vi "Initialize With Options.vi"(7 "option string":string, 8 "error in (no error)":errorcluster {"code" format="%.0x"}, 9 "reset device (Off)":bool, 10 "id query (Off)":bool, 11 "resource string":string caption="resource name") -> (0 "error out":errorcluster {"code" format="%.0x"}, 3 "instrument handle out":refnum<k15>)   [LabVIEW 2014, in "Agilent NA.lvlib"]
doc: "Opens the I/O session to the instrument. Driver methods and properties that access the instrument are only accessible after Initialize is called. Initialize optionally performs a Reset and queries the instrument to validate the instrument model."
uses:
  Agilent NA.lvlib
  AgNA.dll
panel:
  # "© 2014 Agilent Technologies, Inc."
  # "© 2000-2008 National Instruments.  All Rights Reserved."
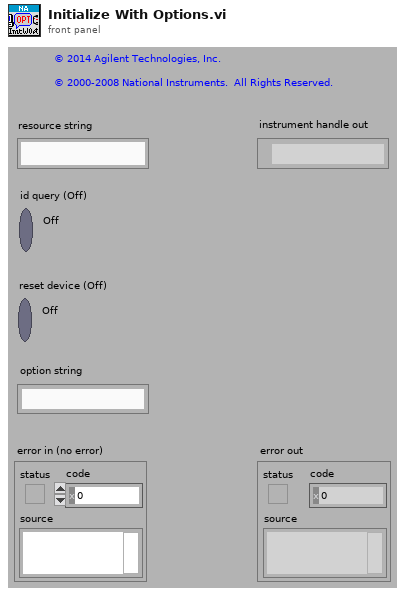
[diagram p1: front panel]
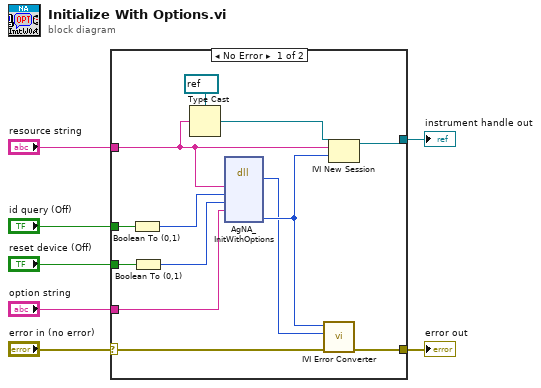
[diagram p0: block diagram]
diagram:
  n1 = case shown="No Error" "error in (no error)" {
    selector: "error in (no error)" -> [w12 w22]
    tunnel: [w11 w22] -> w6
    tunnel: "resource string" -> [w10 w21]
    tunnel: [w18 w21] -> w4
    tunnel: "id query (Off)" -> [w17 _]
    tunnel: "reset device (Off)" -> [w16 _]
    tunnel: "option string" -> [w15 _]
    frame No Error {
      n2 = Boolean To (0,1)(Boolean=w17) -> (0, 1=w20:i16)
      n3 = Boolean To (0,1)(Boolean=w16) -> (0, 1=w19:i16)
      n4 = Type Cast(type=refnum<k15> refnum ("instrument handle out 2"), x=w10) -> (*(type *) &x=w9:refnum<k15>)
      n5 = dll-call lib="AgNA**.dll" fn="AgNA_InitWithOptions" ("LabVIEW:Ivi_InitWithOptionsAndGetError")("resourceDescriptor"=w10, "idQuery"=w20, "reset"=w19, "optionString"=w15) -> ("return type"=w13:i32, "session"=w14:i32)  [unwired: 6 in, 4 out]
      n6 = call "IVI Error Converter.vi"("error in (no error)"=w12, "IVI error code (0)"=w13, "instrument handle"=w14) -> ("error out"=w11:errorcluster)  [unwired: 7 in, 1 out]
      n7 = IVI New Session(9:w14, 10:w10, 11:w9) -> (3:w18:refnum<k15>)
    }
    frame Error {
    }
  }
  "error out" <- w6
  "instrument handle out" <- w4
